vi "Evaluate Name.vi"(10 "Name":string, 11 "Linked List Definition in":refnum<class "Linked List Definition.lvclass">) -> (1 "Match":bool, 2 "Unique ID":string, 3 "Linked List Definition out":refnum<class "Linked List Definition.lvclass">)   [LabVIEW 2017, in "Linked Lists.lvlib" / "Linked List Definition.lvclass"]
uses:
  <vilib>/gpm_packages/@cs/linked-list/Source/Linked List/Linked List Definition/Linked List Definition.lvclass
  <vilib>/gpm_packages/@cs/linked-list/Source/Linked List/Linked List Definition/Linked List Definition.lvclass/Linked List Definition.ctl
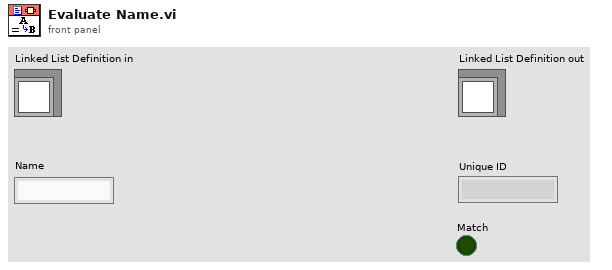
[diagram p1: front panel]
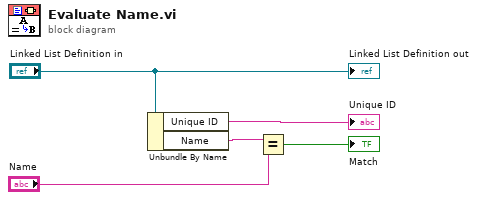
[diagram p0: block diagram]
diagram:
  n1 = Unbundle By Name("Linked List Definition in") -> ("Unique ID"=→"Unique ID":string, "Name"=w4:string)
  n2 = Equal?(x=w4, y="Name") -> (x = y?=→"Match":bool)
  "Linked List Definition out" <- "Linked List Definition in"
